vi "Set Power Level.vi"(8 "error in (no error)":errorcluster, 10 "Power level":dbl, 11 "Electric Fence.lvclass in":refnum<class "Electric Fence.lvclass">) -> (0 "error out":errorcluster, 3 "Electric Fence.lvclass out":refnum<class "Electric Fence.lvclass">)   [LabVIEW 2014, in "Electric Fence.lvclass"]
uses:
  Electric Fence.lvclass
  Electric Fence.lvclass/Electric Fence.ctl
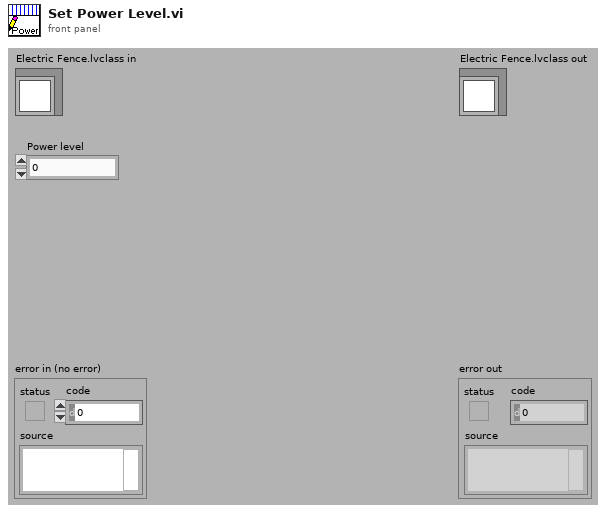
[diagram p1: front panel]
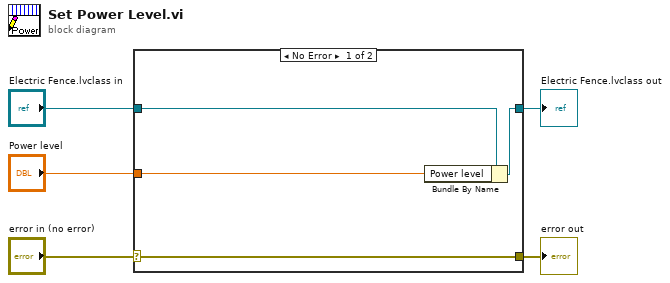
[diagram p0: block diagram]
diagram:
  n1 = case shown="No Error" "error in (no error)" {
    selector: "error in (no error)" -> [w9 w10]
    tunnel: [w9 w10] -> w4
    tunnel: [w7 w11] -> w2
    tunnel: "Electric Fence.lvclass in" -> [w8 w11]
    tunnel: "Power level" -> [w6 _]
    frame No Error {
      n2 = Bundle By Name(cluster=w8, "Power level"=w6) -> (w7:refnum<class "Electric Fence.lvclass">)
    }
    frame Error {
    }
  }
  "error out" <- w4
  "Electric Fence.lvclass out" <- w2
